vi "Error Reported.vi"(8 "error in":errorcluster, 9 "Additional Information":string, 10 "Error":errorcluster, 11 "Module ID":i32=-1) -> (0 "error out":errorcluster)   [LabVIEW 2020, in "Arduino-Adafruit stepper.lvlib"]
doc: "Send the Error Reported event to any VI registered to listen to events from the owning module.\n_____\nBased on DQMH Project Template 7.0.1.1316."
uses:
  Arduino-Adafruit stepper.lvlib
  Error Reported Argument--cluster.ctl
  <vilib>/Delacor/Delacor QMH/Libraries/Message Queue_class/Delacor_lib_QMH_Message Queue.lvclass
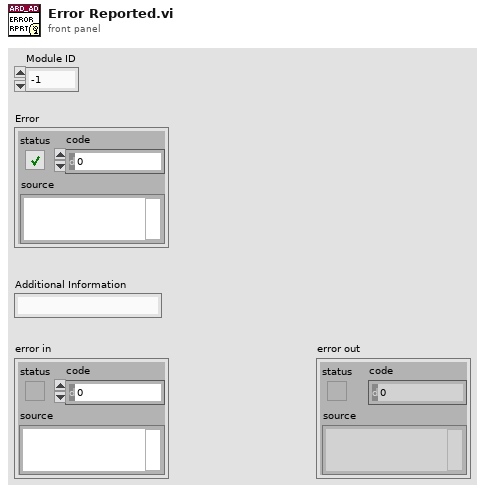
[diagram p1: front panel]
types:
  T1 = typedef "Arduino-Adafruit stepper.lvlib/Error Reported Argument--cluster.ctl" = cluster{"Error":errorcluster, "Additional Information":string, "Module ID":i32, "Module Name":string}
  T2 = typedef "Arduino-Adafruit stepper.lvlib/Broadcast Events--cluster.ctl" = cluster{"Module Did Init":refnum<user-event>, "Status Updated":refnum<user-event>, "Error Reported":refnum<user-event>, "Module Did Stop":refnum<user-event>, "Update Module Execution Status":refnum<user-event>, "Connection successful":refnum<user-event>, "Connection failed":refnum<user-event>, "Device disconnected":refnum<user-event>, "Motors ready":refnum<user-event>, "System busy":refnum<user-event>}
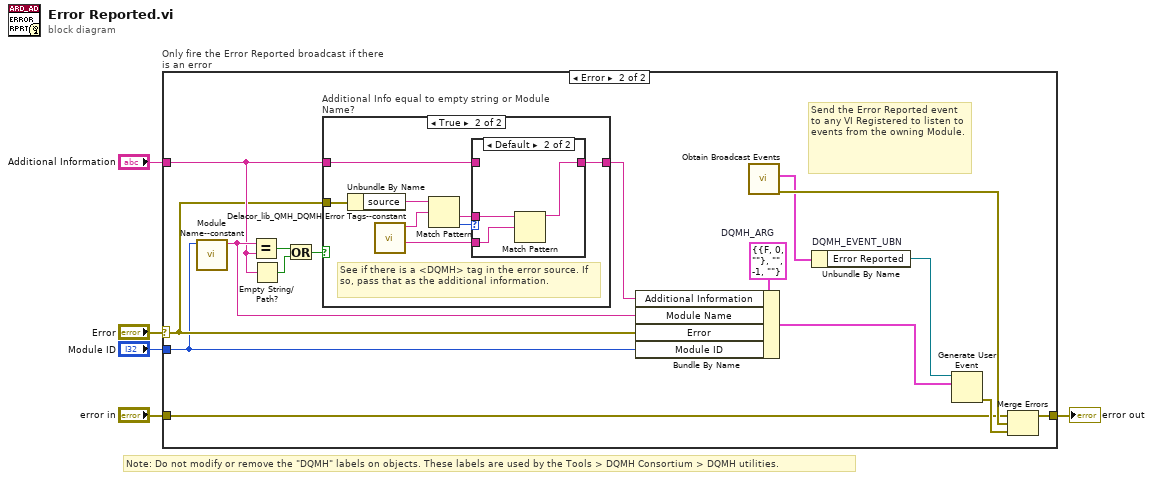
[diagram p0: block diagram]
diagram:
  # "Note: Do not modify or remove the \"DQMH\" labels on objects. These labels are used by the Tools > DQMH Consortium > DQMH utilities."
  n1 = case "Only fire the Error Reported broadcast if there is an error" shown="Error" "Error" {
    selector: "Error" -> [_ w10]
    tunnel: [w6 w22] -> w5
    tunnel: "error in" -> [w6 w7]
    tunnel: "Additional Information" -> [_ w12]
    tunnel: "Module ID" -> [_ w9]
    frame No Error {
      # "No error was wired in, so don't fire the Error Reported broadcast."
    }
    frame Error {
      w18 = T1 {"Error"={"status"=FALSE, "code"=0, "source"=""}, "Additional Information"="", "Module ID"=-1, "Module Name"=""}  # DQMH_ARG
      # "Send the Error Reported event to any VI Registered to listen to events from the owning Module."
      n2 = call "Module Name--constant.vi"("Module ID"=w9) -> ("Module Name"=w16:string)  [unwired: 10 in]
      n3 = Equal?(x=w16, y=w12) -> (x = y?=w15:bool)
      n4 = Empty String/Path?(string/path=w12) -> (empty?=w14:bool)
      n5 = Or(x=w15, y=w14) -> (x .or. y?=w13:bool)
      n6 = case "Additional Info equal to empty string or Module Name?" shown="True" w13 {
        tunnel: w12 -> [w23 w24]
        tunnel: [w23 w25] -> w11
        tunnel: w10 -> [_ w31]
        frame False {
          # "If the additional information string is not equal to empty string or module name, then the user has specified a custom string, and we should pass that value."
        }
        frame True {
          # "See if there is a <DQMH> tag in the error source. If so, pass that as the additional information."
          n7 = Unbundle By Name(w31) -> ("source"=w30:string)
          n8 = call <vilib>:"Delacor_lib_QMH_DQMH Error Tags--constant.vi"() -> ("Close Tag"=w26:string, "Open Tag"=w29:string)  [unwired: 10 in]
          n9 = Match Pattern(string=w30, regular expression=w29) -> (after substring=w27:string, offset past match=w28:i32)  [unwired: 1 in, 2 out]
          n10 = case shown="Default" w28 {
            tunnel: w27 -> [_ w35]
            tunnel: w26 -> [_ w34]
            tunnel: [w32 w33] -> w25
            tunnel: w24 -> [w32 _]
            frame -1 {
            }
            frame Default {
              n11 = Match Pattern(string=w35, regular expression=w34) -> (before substring=w33:string)  [unwired: 1 in, 3 out]
            }
          }
        }
      }
      n12 = Bundle By Name(cluster=w18, "Additional Information"=w11, "Module Name"=w16, "Error"=w10, "Module ID"=w9) -> (w17:T1)
      n13 = call "Obtain Broadcast Events.vi"() -> ("error out"=w21:errorcluster, "Arduino-Adafruit stepper Broadcast Events"=w20:T2)  [unwired: 10 in]
      n14 = Unbundle By Name "DQMH_EVENT_UBN"(w20) -> ("Error Reported"=w19:refnum<user-event>)
      n15 = Generate User Event(user event=w19, event data cluster=w17) -> (error out=w8:errorcluster)  [unwired: 2 in, 1 out]
      n16 = Merge Errors(w7, w21, w8) -> (w22:errorcluster)
    }
  }
  "error out" <- w5
